vi "FTW-Actor-Child-Add.vi"(0 "FTW-ActorExtended In":refnum<class "FTW-ActorInstance.lvclass">, 5 "Identity":string, 7 "Inbox Address":string, 9 "Connection":refnum<class "FTW-ActorConnector.lvclass">, 11 "error in":errorcluster) -> (4 "FTW-ActorExtended Out":refnum<class "FTW-ActorInstance.lvclass">, 15 "error out":errorcluster)   [LabVIEW 2015, in "FTW-ActorInstance.lvclass"]
uses:
  FTW-ActorInstance.lvclass
  Connector/FTW-ActorConnector.lvclass
  FTW-ActorInstance.lvclass/FTW-ActorInstance.ctl
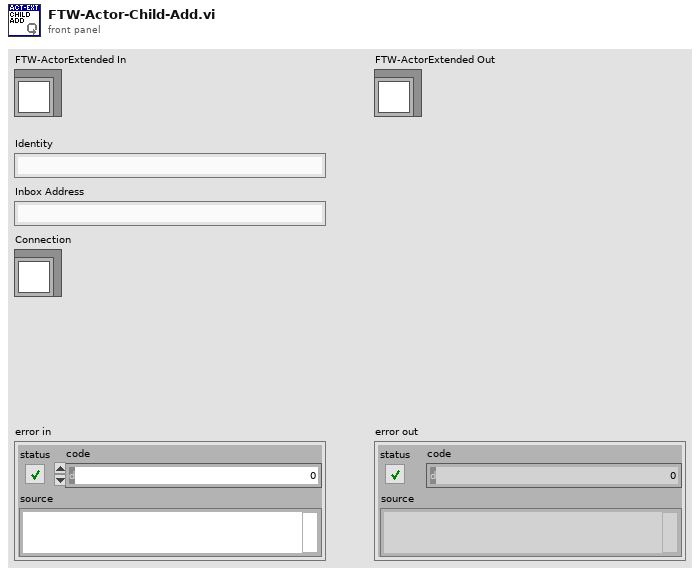
[diagram p1: front panel]
types:
  T1 = cluster{"Identity":string, "Inbox Address":string, "Connection":refnum<class "FTW-ActorConnector.lvclass">, bool}
  T2 = cluster{"Name":string, "URI":string, "Connector":refnum<class "FTW-ActorConnector.lvclass">, "Child":bool}[]
  T3 = cluster{"Identity":string, "Inbox Address":string, "Connection":refnum<class "FTW-ActorConnector.lvclass">, "Child":bool}[]
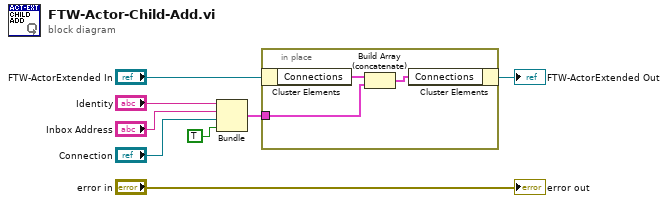
[diagram p0: block diagram]
diagram:
  n1 = Bundle("Identity"="Identity", "Inbox Address"="Inbox Address", "Connection"="Connection", TRUE) -> (w4:T1)  [unwired: 1 in]
  n2 = in-place {
    in-place-border: w4 -> [w9]
    n3 = in-place-cluster #1("FTW-ActorExtended In") -> ("Connections"=w11:T2)
    n4 = Build Array (concatenate)(w11, w9) -> (w10:T3)
    n5 = in-place-cluster #1("Connections"=w10) -> (→"FTW-ActorExtended Out":refnum<class "FTW-ActorInstance.lvclass">)
  }
  "error out" <- "error in"
